vi "intialize picoscope trigger settings.vi"(11 "PicoscopeV2 in":refnum<class "PicoscopeV2.lvclass">) -> (3 "PicoscopeV2 out":refnum<class "PicoscopeV2.lvclass">)   [LabVIEW 2020, in "PicoscopeV2.lvclass"]
uses:
  PicoscopeV2.lvclass
  PicoscopeV2.lvclass/PicoscopeV2.ctl
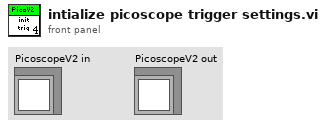
[diagram p1: front panel]
types:
  T1 = enum16{"Channel A", "Channel B", "Channel C", "Channel D", "Ext."}
  T2 = typedef "OnOffTypeDef.ctl" = enum16{"off", "on"}
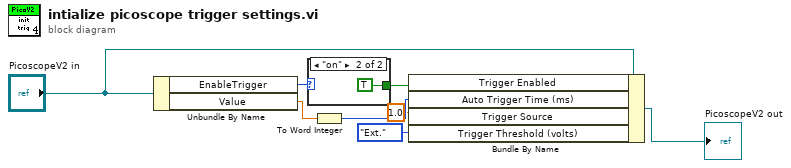
[diagram p0: block diagram]
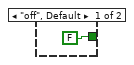
[diagram p2: hidden frame]
diagram:
  n1 = Unbundle By Name("PicoscopeV2 in") -> ("EnableTrigger"=w5:T2, "Value"=w7:dbl)
  n2 = case shown="\"on\"" w5 {
    tunnel: [FALSE TRUE] -> w6
    frame "off", Default {
    }
    frame "on" {
    }
  }
  n3 = To Word Integer(number=w7) -> (16bit integer=w8:i16)
  n4 = Bundle By Name(cluster="PicoscopeV2 in", "Trigger Enabled"=w6, "Auto Trigger Time (ms)"=w8, "Trigger Source"=T1."Ext." ("Trigger Settings.Trigger Source"), "Trigger Threshold (volts)"=1.0 ("Trigger Settings.Trigger Threshold (volts)")) -> (→"PicoscopeV2 out":refnum<class "PicoscopeV2.lvclass">)
